vi "xielu.vi"(5 "waveform in":waveform(dbl)) -> (1 "plot site":cluster{"X":dbl, "Y":dbl}[](array[cluster]), 2 "slop max value":dbl)   [LabVIEW 2011]
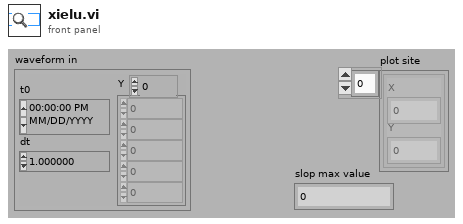
[diagram p1: front panel]
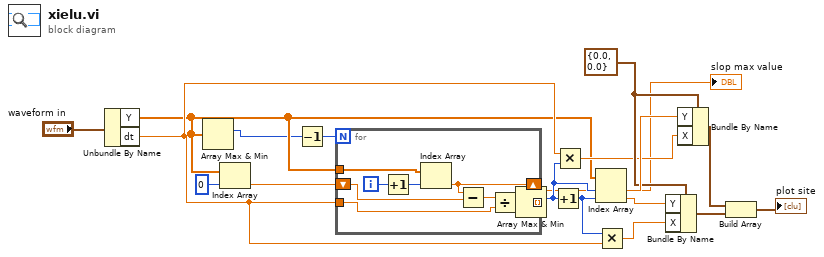
[diagram p0: block diagram]
diagram:
  w13 = cluster{"X":dbl, "Y":dbl} {"X"=0.0, "Y"=0.0}
  n1 = Unbundle By Name("waveform in") -> ("Y"=w3:dbl[], "dt"=w5:dbl)
  n2 = Array Max & Min(array=w3) -> (max index (indices)=w1:i32)  [unwired: 3 out]
  n3 = Index Array(array=w3, index=0) -> (element=w18:dbl)
  n4 = Decrement(x=w1) -> (x-1=w2:i32)
  n5 = for {
    N: w2 -> [_]
    shift-right: [w20] -> _
    shift-left: w18 -> [w27]
    tunnel: w3 -> [w26]
    tunnel: w5 -> [w22]
    tunnel: [w21] -> w17 mode=indexing
    i -> [w24]
    n6 = Increment(x=w24) -> (x+1=w25:i32)
    n7 = Index Array(array=w26, index=w25) -> (element=w20:dbl)
    n8 = Subtract(x=w20, y=w27) -> (x-y=w23:dbl)
    n9 = Divide(x=w23, y=w22) -> (x/y=w21:dbl)
  }
  n10 = Array Max & Min(array=w17) -> (max value=→"slop max value":dbl, max index (indices)=w14:i32)  [unwired: 2 out]
  n11 = Increment(x=w14) -> (x+1=w7:i32)
  n12 = Multiply(x=w5, y=w14) -> (x*y=w6:dbl)
  n13 = Index Array(array=w3, index #1=w14, index #2=w7) -> (element #1=w16:dbl, element #2=w15:dbl)
  n14 = Multiply(x=w7, y=w5) -> (x*y=w8:dbl)
  n15 = Bundle By Name(cluster=w13, "Y"=w15, "X"=w8) -> (w11:cluster{"X":dbl, "Y":dbl})
  n16 = Bundle By Name(cluster=w13, "Y"=w16, "X"=w6) -> (w12:cluster{"X":dbl, "Y":dbl})
  n17 = Build Array(w12, w11) -> (→"plot site":cluster{"X":dbl, "Y":dbl}[])
